vi "ZOH-Inputs.vi"(4 "Plant 2 X2":dbl, 5 "Plant 1 X2":dbl, 6 "Plant 2 X1":dbl, 7 "Plant 1 X1":dbl, 8 "Trigger":bool, 9 "Plant 2 KX Hat":dbl, 10 "Plant 1 KX hat":dbl, 11 "Plant to trigg":enum16{"Plant 1", "Plant 2"}(ring)) -> (1 "Plant 2 KX Hat":dbl, 2 "Plant 1 KX hat":dbl)   [LabVIEW 2016]
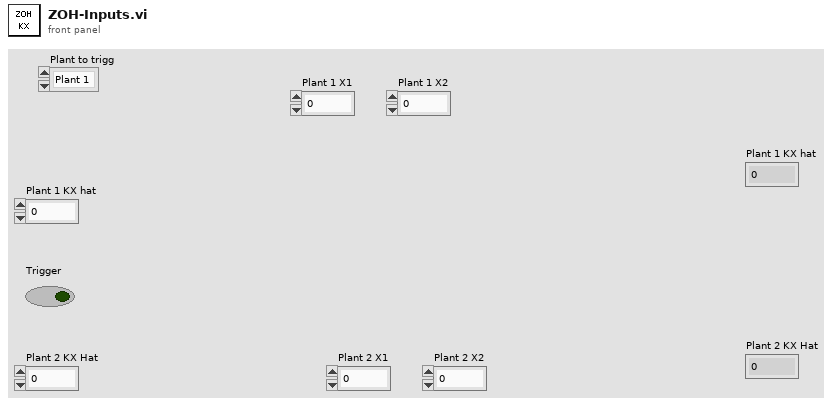
[diagram p1: front panel]
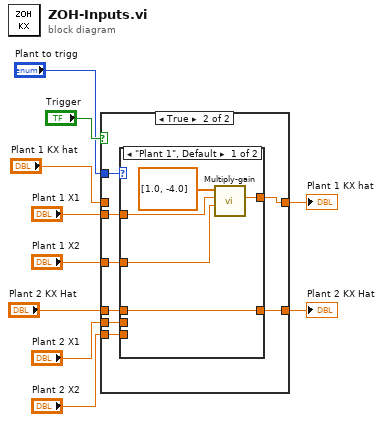
[diagram p0: block diagram]
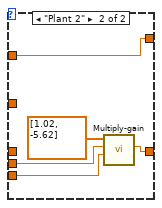
[diagram p3: hidden frame]
diagram:
  n1 = case shown="True" "Trigger" {
    tunnel: "Plant 1 KX hat" -> [w12 _]
    tunnel: "Plant 2 KX Hat" -> [w11 w13]
    tunnel: [w12 w17] -> w7
    tunnel: [w11 w14] -> w6
    tunnel: "Plant to trigg" -> [_ w20]
    tunnel: "Plant 1 X2" -> [_ w19]
    tunnel: "Plant 1 X1" -> [_ w18]
    tunnel: "Plant 2 X1" -> [_ w16]
    tunnel: "Plant 2 X2" -> [_ w15]
    frame False {
    }
    frame True {
      n2 = case shown="\"Plant 1\", Default" w20 {
        tunnel: w19 -> [w25 _]
        tunnel: w18 -> [w24 w30]
        tunnel: [w22 w30] -> w17
        tunnel: w16 -> [_ w28]
        tunnel: w15 -> [_ w27]
        tunnel: [w21 w26] -> w14
        tunnel: w13 -> [w21 _]
        frame "Plant 1", Default {
          n3 = call "Multiply-gain.vi"("X2"=w25, "X1"=w24, "Gain (K)"=dbl[] [1.0, -4.0]) -> ("Kx"=w22:dbl)  [unwired: 8 in]
        }
        frame "Plant 2" {
          n4 = call "Multiply-gain.vi"("X2"=w27, "X1"=w28, "Gain (K)"=dbl[] [1.02, -5.62]) -> ("Kx"=w26:dbl)  [unwired: 8 in]
        }
      }
    }
  }
  "Plant 1 KX hat" <- w7
  "Plant 2 KX Hat" <- w6
